vi "WiFi Thingspeak_SSID.vi"   [LabVIEW 2014]
uses:
  <vilib>/Aledyne-TSXperts/Arduino Compatible Compiler for LabVIEW/Code Generator/Arduino APIs/Digital/PinDirection.ctl
  QwaveSys_ESP8266/QwaveSys_ESP8266.lvlib
  <vilib>/Aledyne-TSXperts/Arduino Compatible Compiler for LabVIEW/Arduino Compatible Compiler for LabVIEW.lvlib
types:
  T1 = typedef "Arduino Compatible Compiler for LabVIEW.lvlib/PinDirection.ctl" = enum16{" INPUT", "OUTPUT", " INPUT_PULLUP"}
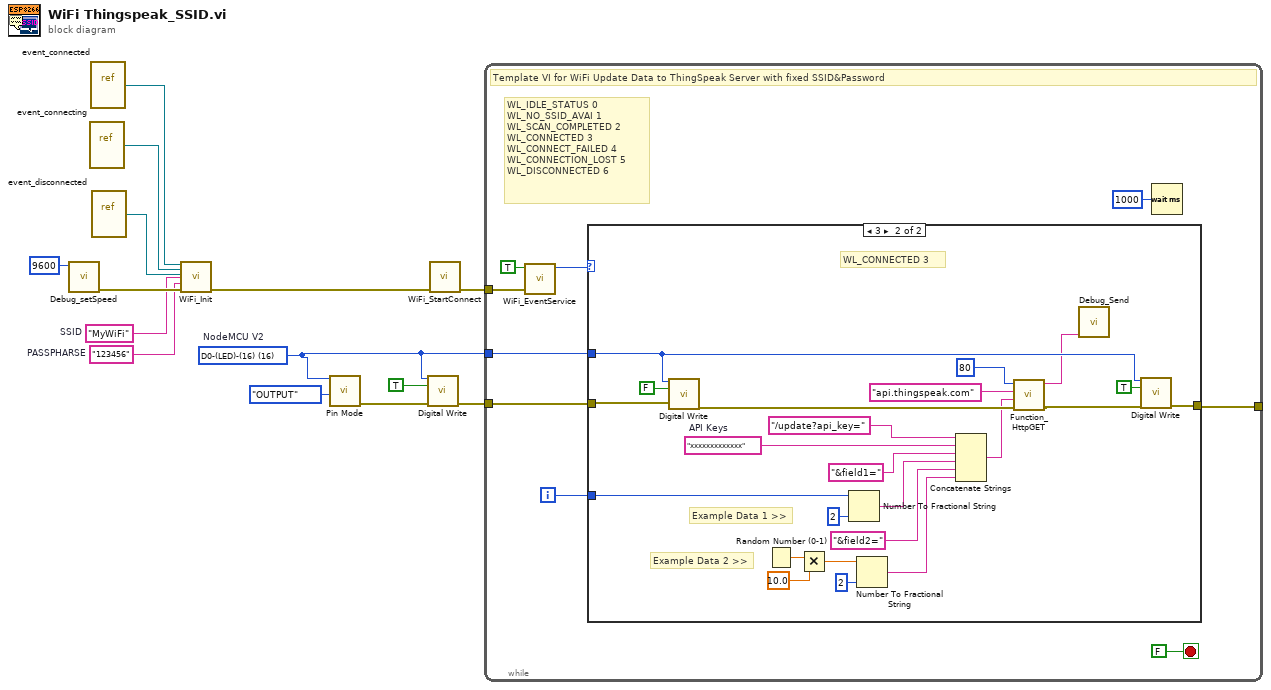
[diagram p0: block diagram]
diagram:
  w1 = u8 16 items=["D0-(LED)-(16)"=16, "D1-SCL(5)"=5, "D2-SDA(4)"=4, "D3-FlashBtn(0)"=0, "D4-(2)"=2, "D5-SCK(14)"=14, "D6-MISO(12)"=12, "D7-MOSI(13)"=13, "D8-SS(15)"=15, "D9-TX(3)"=3, "D10-RX(1)"=1, "ADC0,(17)"=17]  # NodeMCU V2
  w3 = "123456"  # PASSPHARSE
  w4 = "MyWiFi"  # SSID
  n1 = call "Debug_setSpeed.vi"("Speed"=u32 9600) -> ("error out"=w10:errorcluster)  [unwired: 10 in]
  n2 = vi-ref "event_connecting.vi"() -> (w13:refnum<vi>)
  n3 = vi-ref "event_connected.vi"() -> (w12:refnum<vi>)
  n4 = vi-ref "event_disconnected.vi"() -> (w11:refnum<vi>)
  n5 = call "WiFi_Init.vi"("connected"=w12, "connecting"=w13, "disconnected"=w11, "SSID"=w4, "PASSPHARSE"=w3, "error in (no error)"=w10) -> ("error out"=w2:errorcluster)  [unwired: 9 in]
  n6 = call <vilib>:"Pin Mode.vi"("pin"=w1, "direction"=PinDirection."OUTPUT") -> ("error out"=w7:errorcluster)  [unwired: 13 in]
  n7 = call <vilib>:"Digital Write.vi"("pin"=w1, "state"=TRUE, "error in (no error)"=w7) -> ("error out"=w5:errorcluster)  [unwired: 12 in]
  n8 = call "WiFi_StartConnect.vi"("error in (no error)"=w2) -> ("error out"=w14:errorcluster)  [unwired: 10 in]
  n9 = while {
    tunnel: w14 -> [w22]
    tunnel: w5 -> [w18]
    tunnel: w1 -> [w17]
    tunnel: [w15] -> _
    i -> [w16]
    stop <- FALSE stop-if-true
    # "WL_IDLE_STATUS\t0\nWL_NO_SSID_AVAI\t1\nWL_SCAN_COMPLETED\t2\nWL_CONNECTED\t3\nWL_CONNECT_FAILED\t4\nWL_CONNECTION_LOST\t5\nWL_DISCONNECTED\t6"
    # "Template VI for WiFi Update Data to ThingSpeak Server with fixed SSID&Password"
    n10 = call "WiFi_EventService.vi"("error in (no error)"=w22, "wait for connected (True)"=TRUE) -> ("Status"=w19:u16)  [unwired: 8 in, 1 out]
    n11 = case shown="3" w19 {
      tunnel: w18 -> [w24 w31]
      tunnel: w17 -> [_ w29]
      tunnel: w16 -> [_ w28]
      tunnel: [w24 w27] -> w15
      frame 0, Default {
        # "DISCONNECTED or default status"
      }
      frame 3 {
        w33 = "xxxxxxxxxxxxx"  # API Keys
        # "Example Data 2 >>"
        # "Example Data 1 >>"
        # "WL_CONNECTED\t3"
        n12 = call <vilib>:"Digital Write.vi"("pin"=w29, "state"=FALSE, "error in (no error)"=w31) -> ("error out"=w44:errorcluster)  [unwired: 12 in]
        n13 = Random Number (0-1)() -> (number: 0 to 1=w40:dbl)
        n14 = Multiply(x=w40, y=10.0) -> (x*y=w41:dbl)
        n15 = Number To Fractional String(number=w28, precision (6)=i16 2) -> (F-format string=w37:string)  [unwired: 2 in]
        n16 = Number To Fractional String(number=w41, precision (6)=i16 2) -> (F-format string=w43:string)  [unwired: 2 in]
        n17 = Concatenate Strings("/update?api_key=", w33, "&field1=", w37, "&field2=", w43) -> (w34:string)
        n18 = call "Function_HttpGET.vi"("error in (no error)"=w44, "URI"=w34, "Host"="api.thingspeak.com", "Port"=i8 80) -> ("error out"=w26:errorcluster, "Results"=w25:string)  [unwired: 6 in]
        n19 = call "Debug_Send.vi"("DATA"=w25) -> ()  [unwired: 11 in]
        n20 = call <vilib>:"Digital Write.vi"("pin"=w29, "state"=TRUE, "error in (no error)"=w26) -> ("error out"=w27:errorcluster)  [unwired: 12 in]
      }
    }
    n21 = Wait (ms)(milliseconds to wait=u32 1000) -> ()  [unwired: 1 out]
  }
